vi "get stream meta channels.vi"(8 "error in":errorcluster, 11 "stream ref in":T2 format="%.0x") -> (0 "error out":errorcluster, 1 "status (out) channel":T2 format="%.0x", 2 "decimation (in) channel":T2 format="%.0x", 3 "enable (in) channel":T2 format="%.0x", 5 "time (in) channel":T2 format="%.0x", 7 "time source":T1)   [LabVIEW 2026, in "Nominal Core Streaming Shared.lvlib"]
uses:
  Nominal Core Streaming Shared.lvlib
  <vilib>/NI VeriStand/Custom Device API/Custom Device Item Ref.ctl
  time convert type.ctl
  Constants.vi
  <vilib>/NI VeriStand/Custom Device Tools/Custom Device Utility Library/Custom Device Utility Library.lvlib
  <vilib>/NI VeriStand/Custom Device API/Custom Device API.lvlib
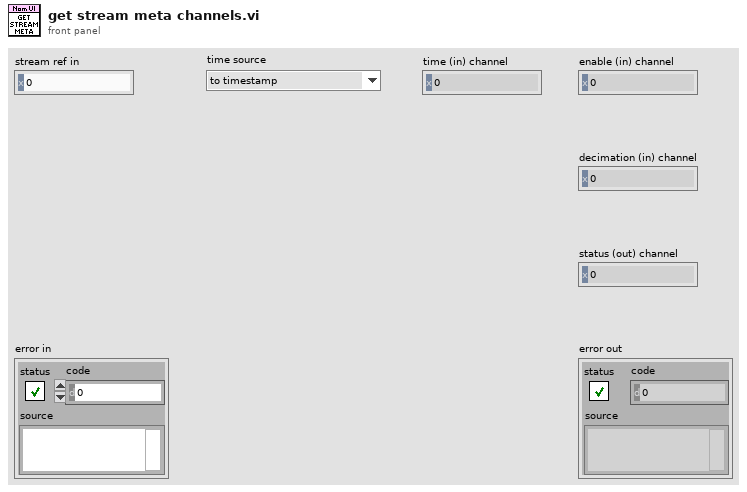
[diagram p1: front panel]
types:
  T1 = typedef "Nominal Core Streaming Shared.lvlib/time convert type.ctl" = enum16{"to timestamp", "relative seconds"}
  T2 = typedef "Custom Device API.lvlib/Custom Device Item Ref.ctl" = u64
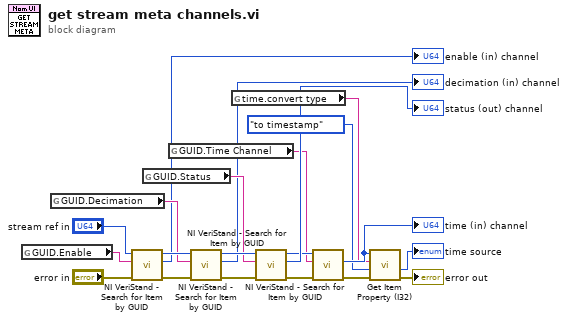
[diagram p0: block diagram]
diagram:
  n1 = global read "Constants.vi" "GUID.Enable"() -> (w14:string)
  n2 = global read "Constants.vi" "GUID.Decimation"() -> (w15:string)
  n3 = call <vilib>:"NI VeriStand - Search for Item by GUID.vi"("error in"="error in", "Item GUID"=w14, "Section Ref in"="stream ref in") -> ("error out"=w21:errorcluster, "Item Ref"=→"enable (in) channel":T2, "Section Ref out"=w20:T2)  [unwired: 5 in, 1 out]
  n4 = global read "Constants.vi" "GUID.Status"() -> (w16:string)
  n5 = global read "Constants.vi" "GUID.Time Channel"() -> (w7:string)
  n6 = call <vilib>:"NI VeriStand - Search for Item by GUID.vi"("error in"=w21, "Item GUID"=w15, "Section Ref in"=w20) -> ("error out"=w19:errorcluster, "Item Ref"=→"decimation (in) channel":T2, "Section Ref out"=w18:T2)  [unwired: 5 in, 1 out]
  n7 = global read "Constants.vi" "time.convert type"() -> (w3:string)
  n8 = call <vilib>:"NI VeriStand - Search for Item by GUID.vi"("error in"=w19, "Item GUID"=w16, "Section Ref in"=w18) -> ("error out"=w9:errorcluster, "Item Ref"=→"status (out) channel":T2, "Section Ref out"=w8:T2)  [unwired: 5 in, 1 out]
  n9 = call <vilib>:"NI VeriStand - Search for Item by GUID.vi"("error in"=w9, "Item GUID"=w7, "Section Ref in"=w8) -> ("error out"=w6:errorcluster, "Item Ref"=w4:T2)  [unwired: 5 in, 2 out]
  "time (in) channel" <- w4
  n10 = call <vilib>:"Get Item Property (I32).vi"("error in (no error)"=w6, "Default Value"=time_convert_type."to timestamp" ("time source"), "Property Name"=w3, "Item Ref in"=w4) -> ("error out"=→"error out":errorcluster, "Value"=→"time source":i32)  [unwired: 4 in, 2 out]
